vi "Create DO Channel Wrapper.vi"(0 "Task map in":map{string, refnum<k21>}(c390), 5 "Message Data in":T2, 11 "error in (no error)":errorcluster) -> (4 "Task map out":map{string, refnum<k21>}(c390), 6 "Message Data out":T1, 15 "error out":errorcluster)   [LabVIEW 2021, in "NI DAQmx_wrapper.lvlib"]
uses:
  NI DAQmx_wrapper.lvlib
  NI DAQmx_server/RPC Messages/nidaqmx_grpc_CreateDOChanRequest.ctl
  NI DAQmx_server/RPC Messages/nidevice_grpc_Session_session/nidevice_grpc_Session_session.lvclass
  NI DAQmx_server/RPC Messages/nidaqmx_grpc_CreateDOChanRequest_line_grouping_enum/nidaqmx_grpc_CreateDOChanRequest_line_grouping_enum.lvclass
  NI DAQmx_server/RPC Messages/nidevice_grpc_Session.ctl
  NI DAQmx_server/RPC Messages/nidaqmx_grpc_CreateDOChanResponse.ctl
  NI DAQmx_server/RPC Messages/nidaqmx_grpc_CreateDOChanRequest_line_grouping_enum/nidaqmx_grpc_CreateDOChanRequest_line_grouping_enum.lvclass/nidaqmx_grpc_CreateDOChanRequest_line_grouping_enum.ctl
  NI DAQmx_server/RPC Messages/nidevice_grpc_Session_session/nidevice_grpc_Session_session.lvclass/nidevice_grpc_Session_session.ctl
  <vilib>/DAQmx/create/channels.llb/DAQmx Create Channel (DO-Digital Output).vi
  NI DAQmx_server/NI DAQmx_server.lvlib
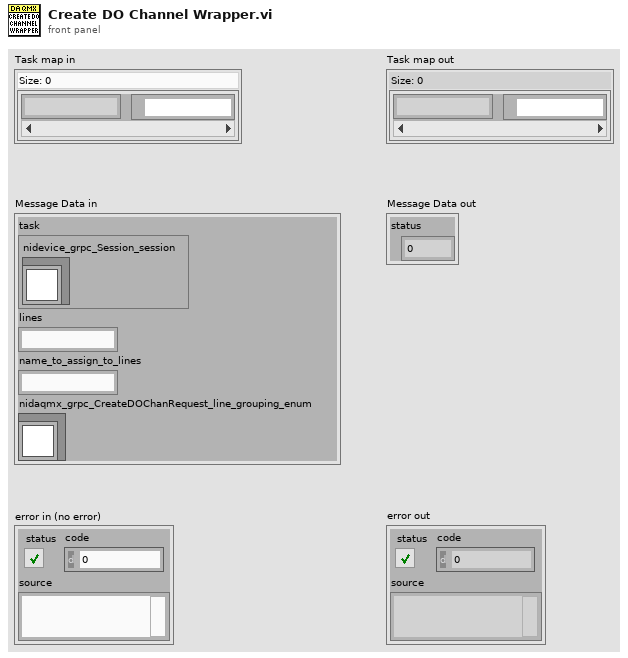
[diagram p1: front panel]
types:
  T1 = typedef "NI DAQmx_server.lvlib/nidaqmx_grpc_CreateDOChanResponse.ctl" = cluster{"status":i32}
  T2 = typedef "NI DAQmx_server.lvlib/nidaqmx_grpc_CreateDOChanRequest.ctl" = cluster{"task":T3, "lines":string, "name_to_assign_to_lines":string, "nidaqmx_grpc_CreateDOChanRequest_line_grouping_enum":refnum<class "nidaqmx_grpc_CreateDOChanRequest_line_grouping_enum.lvclass">}
  T3 = typedef "NI DAQmx_server.lvlib/nidevice_grpc_Session.ctl" = cluster{"nidevice_grpc_Session_session":refnum<class "nidevice_grpc_Session_session.lvclass">}
  T4 = typedef "NI DAQmx_server.lvlib/nidaqmx_grpc_LineGrouping.ctl" = enum32{"LINE_GROUPING_CHAN_PER_LINE", "LINE_GROUPING_CHAN_FOR_ALL_LINES"}
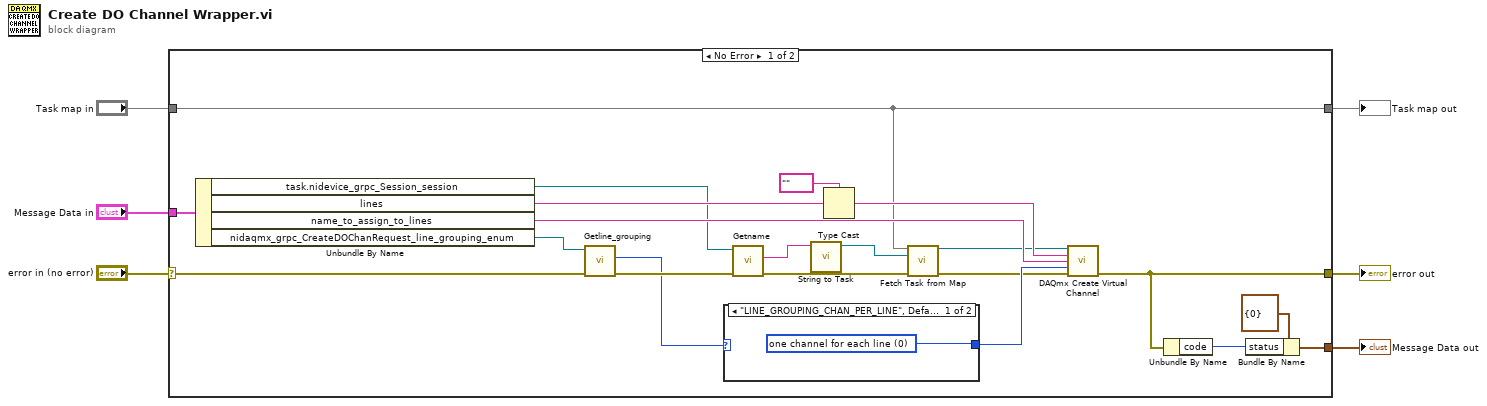
[diagram p0: block diagram]
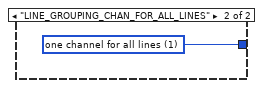
[diagram p2: hidden frame]
diagram:
  n1 = case shown="No Error" "error in (no error)" {
    selector: "error in (no error)" -> [w20 w31]
    tunnel: [w11 w31] -> w5
    tunnel: [w14 w30] -> w3
    tunnel: "Task map in" -> [w14 w30]
    tunnel: "Message Data in" -> [w27 _]
    tunnel: [w7 _] -> w1
    frame No Error {
      n2 = Unbundle By Name(w27) -> ("task.nidevice_grpc_Session_session"=w10:refnum<class "nidevice_grpc_Session_session.lvclass">, "lines"=w25:string, "name_to_assign_to_lines"=w22:string, "nidaqmx_grpc_CreateDOChanRequest_line_grouping_enum"=w21:refnum<class "nidaqmx_grpc_CreateDOChanRequest_line_grouping_enum.lvclass">)
      n3 = call "Getline_grouping.vi"("error in (no error)"=w20, "OneOfTemplate in"=w21) -> ("error out"=w19:errorcluster, "Get_Val"=w18:T4)  [unwired: 7 in, 1 out]
      n4 = case shown="\"LINE_GROUPING_CHAN_PER_LINE\", Default" w18 {
        tunnel: [w28 w29] -> w17
        frame "LINE_GROUPING_CHAN_PER_LINE", Default {
          w28 = 0 items=["one channel for each line", "one channel for all lines"] ("line grouping")
        }
        frame "LINE_GROUPING_CHAN_FOR_ALL_LINES" {
          w29 = 1 items=["one channel for each line", "one channel for all lines"] ("line grouping")
        }
      }
      n5 = call "Getname.vi"("error in (no error)"=w19, "OneOfTemplate in"=w10) -> ("error out"=w16:errorcluster, "Get_Val"=w26:string)  [unwired: 7 in, 1 out]
      n6 = call "String to Task.vi"("Get_Val"=w26) -> ("Refnum out"=w13:refnum<k21>)  [unwired: 10 in]
      n7 = Type Cast(type=tag "" ("lines"), x=w25) -> (*(type *) &x=w23:tag)
      n8 = call "Fetch Task from Map.vi"("Task map in"=w14, "Task in"=w13, "error in (no error)"=w16) -> ("Task out"=w12:refnum<k21>, "error out"=w15:errorcluster)  [unwired: 10 in, 1 out]
      n9 = call-poly <vilib>:"DAQmx Create Virtual Channel.vi"("task in"=w12, "lines"=w23, "name to assign"=w22, "line grouping"=w17, "error in"=w15) -> ("error out"=w11:errorcluster)  [unwired: 9 in, 1 out]
      n10 = Unbundle By Name(w11) -> ("code"=w8:i32)
      n11 = Bundle By Name(cluster=T1 {"status"=0} ("Message Data out"), "status"=w8) -> (w7:T1)
    }
    frame Error {
    }
  }
  "error out" <- w5
  "Task map out" <- w3
  "Message Data out" <- w1
